vi "SLSC Read Capabilities File from Disk_O2.vi"(8 "error in (no error)":errorcluster) -> (0 "error out":errorcluster, 3 "String":string)   [LabVIEW 2017]
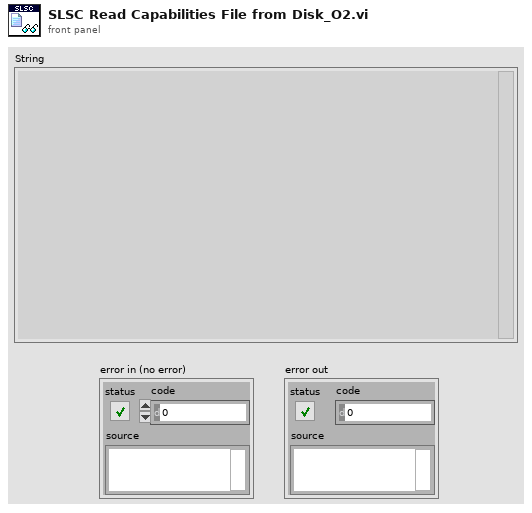
[diagram p1: front panel]
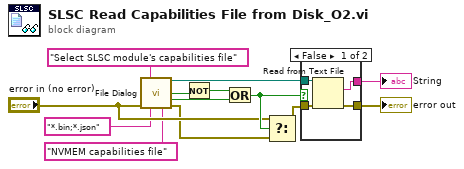
[diagram p0: block diagram]
diagram:
  n1 = call "File Dialog"("prompt"="Select SLSC module's capabilities file", "error in"="error in (no error)", "pattern (all files)"="*.bin;*.json", "pattern label"="NVMEM capabilities file") -> ("selected path"=w3:path, "exists"=w11:bool, "cancelled"=w7:bool, "error out"=w8:errorcluster)  [unwired: 8 in]
  n2 = Not(x=w11) -> (.not. x?=w10:bool)
  n3 = Or(x=w10, y=w7) -> (x .or. y?=w13:bool)
  n4 = Select(t="error in (no error)", s=w13, f=w8) -> (s? t:f=w9:errorcluster)
  n5 = case shown="False" w13 {
    tunnel: w3 -> [w17 _]
    tunnel: [w16 w18] -> w4
    tunnel: [w15 _] -> w5
    tunnel: w9 -> [w14 w18]
    frame False {
      n6 = Read from Text File(file (use dialog)=w17, error in=w14) -> (text=w15:string, error out=w16:errorcluster)  [unwired: 2 in, 2 out]
    }
    frame True {
    }
  }
  "String" <- w5
  "error out" <- w4
